vi "Enqueue in Middle.vi"(8 "error in (no error)":errorcluster, 10 "Array":string[](array[string]), 11 "Queue in":refnum<queue>) -> (0 "error out":errorcluster)   [LabVIEW 2019]
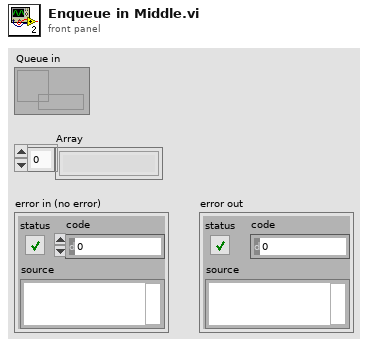
[diagram p1: front panel]
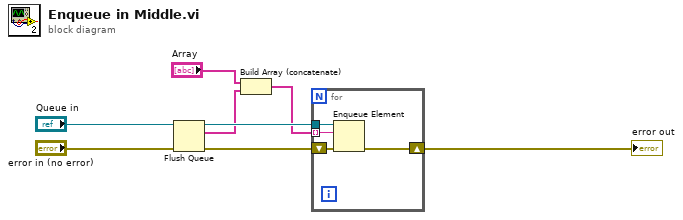
[diagram p0: block diagram]
diagram:
  n1 = Flush Queue(queue="Queue in", error in (no error)="error in (no error)") -> (queue out=w4:refnum<queue>, remaining elements=w2:string[], error out=w6:errorcluster)
  n2 = Build Array (concatenate)("Array", w2) -> (w1:string[])
  n3 = for {
    shift-right: [w11] -> w8
    shift-left: w6 -> [w12]
    tunnel: w4 -> [w10]
    tunnel: w1 -> [w9] mode=indexing
    n4 = Enqueue Element(queue=w10, element=w9, error in (no error)=w12) -> (error out=w11:errorcluster)  [unwired: 1 in, 2 out]
  }
  "error out" <- w8
